vi "(SubVI) Calculate window frame BM.vi"(4 "Window BM":i32=30, 5 "nm/pixel":dbl, 6 "all x position (pixel)":dbl[](array[numeric])) -> (1 "BM":dbl[](array[numeric]), 2 "sec":dbl[](array[numeric]), 3 "frame":i32)   [LabVIEW 2016]
uses:
  <vilib>/Analysis/NI_AALBase.lvlib
panel:
  out "Fs (Hz)":dbl=30.0
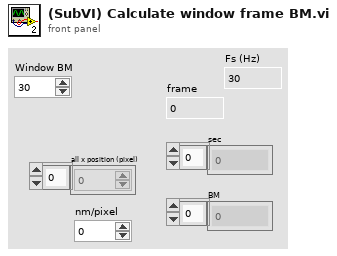
[diagram p1: front panel]
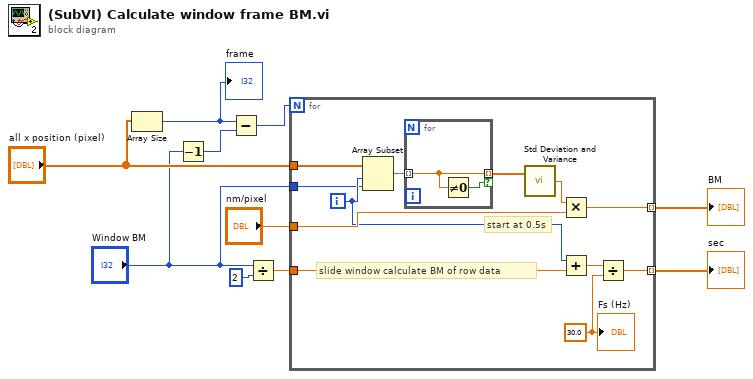
[diagram p0: block diagram]
diagram:
  n1 = Array Size(array="all x position (pixel)") -> (size(s)=w7:i32)
  "frame" <- w7
  n2 = Decrement(x="Window BM") -> (x-1=w4:i32)
  n3 = Subtract(x=w7, y=w4) -> (x-y=w6:i32)
  n4 = Divide(x="Window BM", y=2) -> (x/y=w1:dbl)
  n5 = for {
    N: w6 -> [_]
    tunnel: "all x position (pixel)" -> [w15]
    tunnel: [w19] -> w9 mode=indexing
    tunnel: [w20] -> w10 mode=indexing
    tunnel: "nm/pixel" -> [w18]
    tunnel: "Window BM" -> [w12]
    tunnel: w1 -> [w17]
    i -> [w14]
    w16 = 30.0 ("y")
    # "start at 0.5s"
    # "slide window calculate BM of row data"
    n6 = Array Subset(array=w15, index=w14, length=w12) -> (w13:dbl[])
    n7 = for {
      tunnel: w13 -> [w24] mode=indexing
      tunnel: [w24] -> w11 mode=indexing if=w23
      n8 = Not Equal To 0?(x=w24) -> (x != 0?=w23:bool)
    }
    n9 = call <vilib>:"Std Deviation and Variance.vi"("X"=w11) -> ("standard deviation"=w22:dbl)  [unwired: 1 in, 2 out]
    n10 = Multiply(x=w22, y=w18) -> (x*y=w19:dbl)
    n11 = Add(x=w14, y=w17) -> (x+y=w21:dbl)
    n12 = Divide(x=w21, y=w16) -> (x/y=w20:dbl)
    "Fs (Hz)" <- w16
  }
  "sec" <- w10
  "BM" <- w9
